vi "simple_acc_test.vi"() -> ()   [LabVIEW 2013]
uses:
  <vilib>/Analysis/2dsp.llb/Integral Method.ctl
  <vilib>/Analysis/8numeric.llb/1D Numeric Integration.vi
  <vilib>/Analysis/NI_AALPro.lvlib
panel:
  out "웨이브폼 차트":dbl(graph)
  in  "불리언":bool
  out "result":dbl caption="적분값" format="%0.4f"
  out "dt":dbl
  out "9215":waveform(dbl)(graph)
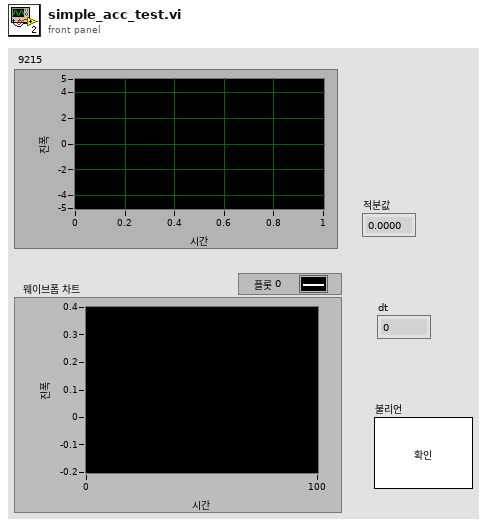
[diagram p1: front panel]
types:
  T1 = typedef "NI_AALPro.lvlib/Integral Method.ctl" = i32
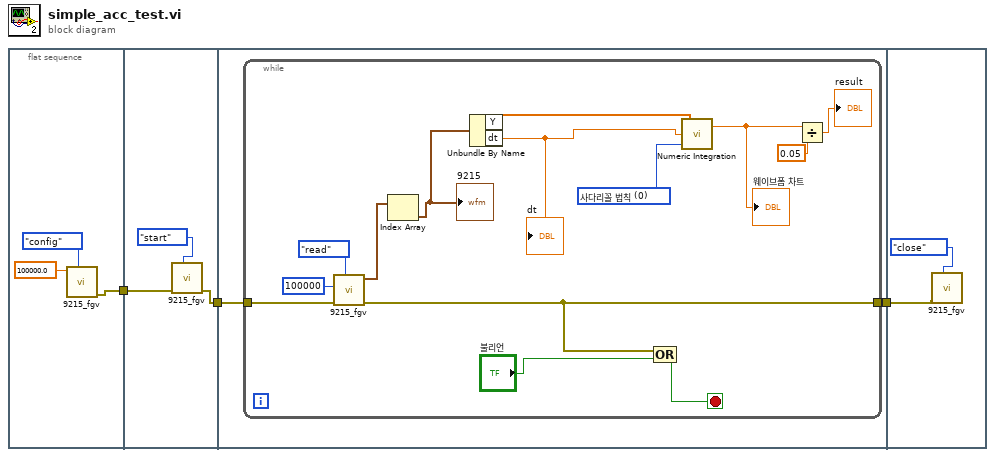
[diagram p0: block diagram]
diagram:
  n1 = flat-sequence {
    tunnel: [w4] -> w3
    tunnel: w3 -> [w8]
    tunnel: [w7] -> w2
    tunnel: w2 -> [w11]
    tunnel: [w10] -> w1
    tunnel: w1 -> [w26]
    frame #0 {
      n2 = call "9215_fgv.vi"("cmd"=enum16{"config", "start", "read", "close"}."config", "rate"=100000.0) -> ("error out"=w4:errorcluster)  [unwired: 8 in, 1 out]
    }
    frame #1 {
      n3 = call "9215_fgv.vi"("cmd"=enum16{"config", "start", "read", "close"}."start", "error in"=w8) -> ("error out"=w7:errorcluster)  [unwired: 8 in, 1 out]
    }
    frame #2 {
      n4 = while {
        tunnel: w11 -> [w23]
        tunnel: [w20] -> w10
        stop <- w21 stop-if-true
        w19 = T1 0 items=["사다리꼴 법칙", "심슨의 법칙", "심슨의 3/8 법칙", "보데 법칙"] ("integration method")
        n5 = call "9215_fgv.vi"("cmd"=enum16{"config", "start", "read", "close"}."read", "error in"=w23, "number of samples per channel"=100000) -> ("error out"=w20:errorcluster, "data"=w22:waveform(dbl)[])  [unwired: 7 in]
        n6 = Index Array(array=w22) -> (element=w18:waveform(dbl))  [unwired: 1 in]
        "9215" <- w18
        n7 = Unbundle By Name(w18) -> ("Y"=w16:dbl[], "dt"=w17:dbl)
        "dt" <- w17
        n8 = Compound Arithmetic op=OR(w20, "불리언") -> (w21:bool)
        n9 = call-poly <vilib>:"Numeric Integration.vi"("integration method"=w19, "dt"=w17, "Input Array"=w16) -> ("result"=w14:dbl)  [unwired: 1 out]
        "웨이브폼 차트" <- w14
        n10 = Divide(x=w14, y=0.05) -> (x/y=→"result":dbl)
      }
    }
    frame #3 {
      n11 = call "9215_fgv.vi"("cmd"=enum16{"config", "start", "read", "close"}."close", "error in"=w26) -> ()  [unwired: 8 in, 2 out]
    }
  }
